vi "Fibonacci series.vi"(3 "Generate Fibonacci terms that are <= this number (dflt=one million)":u64=1000000) -> (0 "Number of elements in series":i32, 1 "Fibonacci series":u64[](array[numeric]))   [LabVIEW 2021, in "Numeric Utilities.lvlib"]
uses:
  Numeric Utilities.lvlib
panel:
  out "Current Fibonacci term":u64
  # "Development\ncontrols/indicators useful for development and testing, but which are not outputs of the VI"
  # "Input\nInputs to the VI"
  # "Output\nOutputs of the VI"
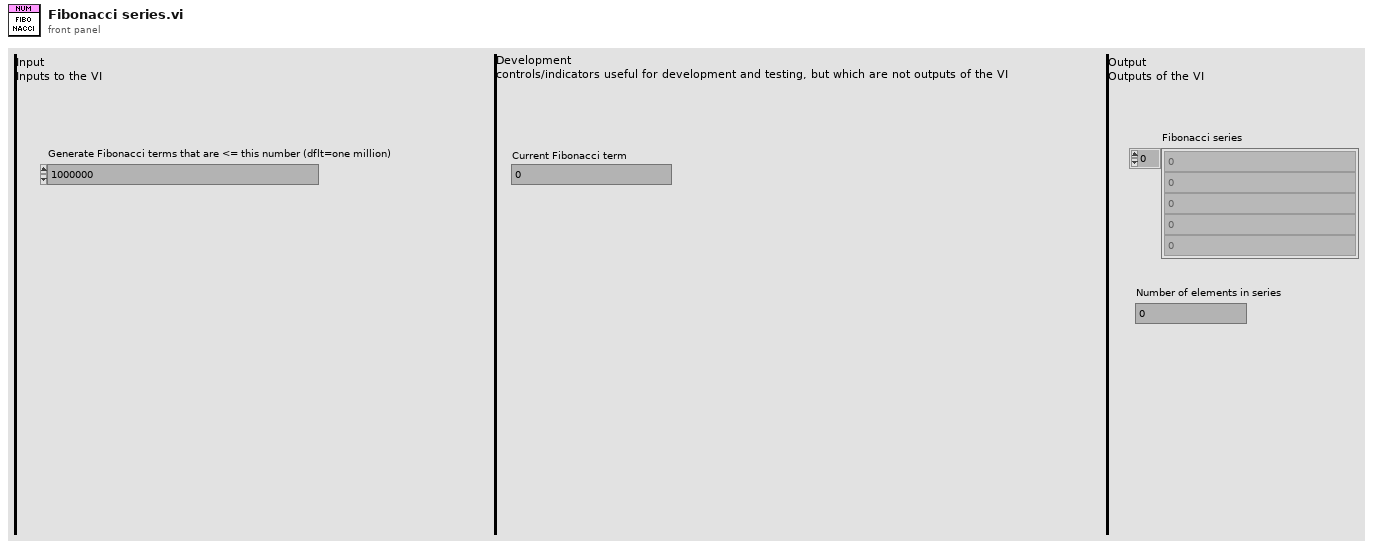
[diagram p1: front panel]
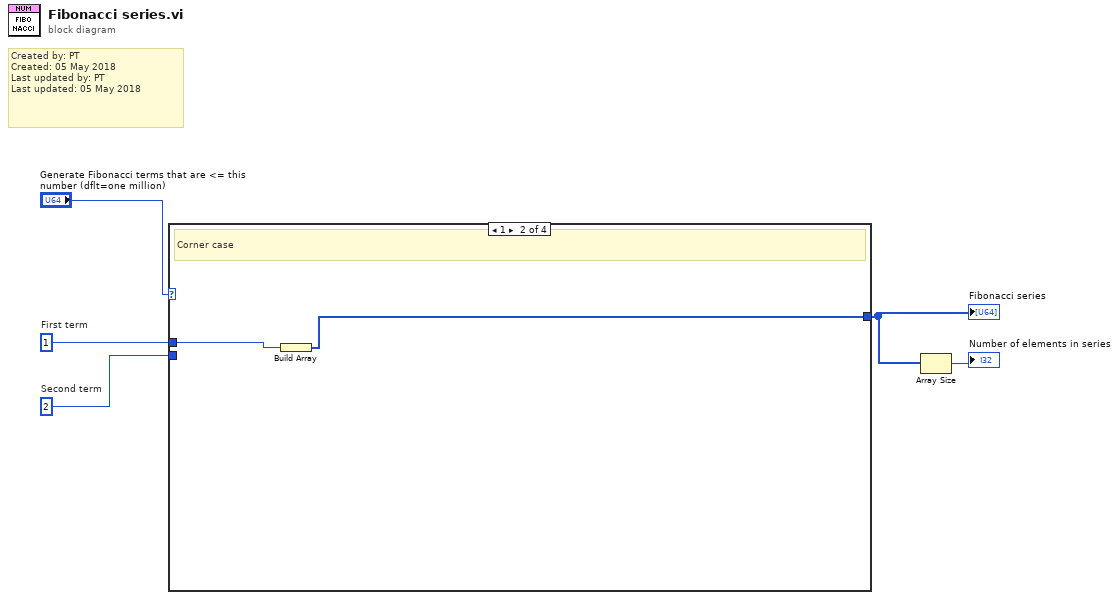
[diagram p0: block diagram]
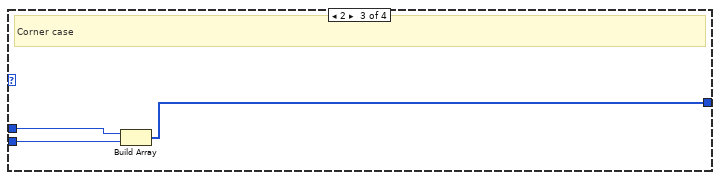
[diagram p3: hidden frame]
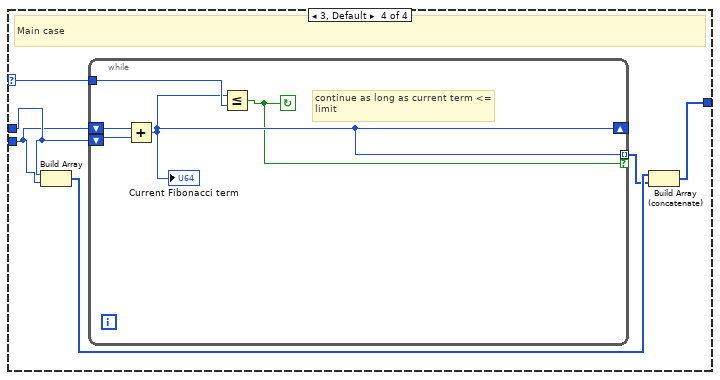
[diagram p4: hidden frame]
diagram:
  w1 = u64 2  # Second term
  w2 = u64 1  # First term
  # "Created by: PT\nCreated: 05 May 2018\nLast updated by: PT\nLast updated: 05 May 2018"
  n1 = case shown="1" "Generate Fibonacci terms that are <= this number (dflt=one million)" {
    selector: "Generate Fibonacci terms that are <= this number (dflt=one million)" -> [_ _ _ w16]
    tunnel: [_ w6 w9 w11] -> w4
    tunnel: w2 -> [_ w7 w10 w15]
    tunnel: w1 -> [_ _ w8 w14]
    frame 0 {
      # "Corner case: user requests Fibonacci terms <= 0. Return empty series."
    }
    frame 1 {
      # "Corner case"
      n2 = Build Array(w7) -> (w6:u64[])
    }
    frame 2 {
      # "Corner case"
      n3 = Build Array(w10, w8) -> (w9:u64[])
    }
    frame 3, Default {
      # "Main case"
      n4 = Build Array(w15, w14) -> (w13:u64[])
      n5 = while {
        tunnel: w16 -> [w21]
        shift-right: [w18] -> _
        shift-left: w14 -> [w20]
        shift-left: w15 -> [w19]
        tunnel: [w18] -> w12 mode=indexing if=w17
        stop <- w17 continue-if-true
        # "continue as long as current term <= limit"
        n6 = Add(x=w20, y=w19) -> (x+y=w18:u64)
        "Current Fibonacci term" <- w18
        n7 = Less Or Equal?(x=w18, y=w21) -> (x <= y?=w17:bool)
      }
      n8 = Build Array (concatenate)(w13, w12) -> (w11:u64[])
    }
  }
  "Fibonacci series" <- w4
  n9 = Array Size(array=w4) -> (size(s)=→"Number of elements in series":i32)
